vi "Get LabVIER Version.vi"(8 "错误输入（无错误）":errorcluster) -> (0 "错误输出":errorcluster, 3 "输出簇":T1)   [LabVIEW 2012, in "Application.lvlib"]
uses:
  Application.lvlib
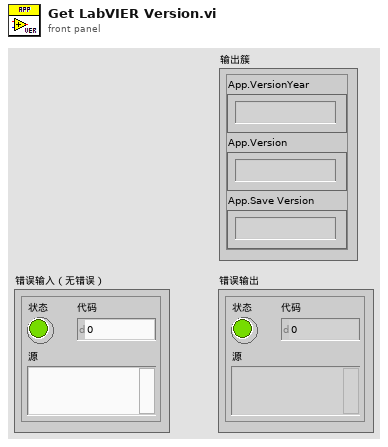
[diagram p1: front panel]
types:
  T1 = cluster{"App.VersionYear":string, "App.Version":string, "App.Save Version":string}
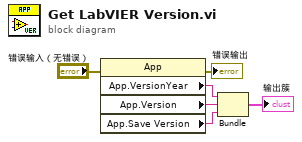
[diagram p0: block diagram]
diagram:
  n1 = property class="App"(error in="错误输入（无错误）") -> (error out=→"错误输出":errorcluster, "App.VersionYear"=w6:string, "App.Version"=w5:string, "App.Save Version"=w4:string)  [unwired: 1 in, 1 out]
  n2 = Bundle("App.VersionYear"=w6, "App.Version"=w5, "App.Save Version"=w4) -> (→"输出簇":T1)  [unwired: 1 in]
